vi "Write Ch 02.vi"(8 "error in":errorcluster, 10 "Producer Ch 02":T1, 11 "Chiller Cluster - 2 Channel.lvclass":refnum<class "Chiller Cluster - 2 Channel.lvclass">) -> (0 "error out":errorcluster, 3 "output cluster":refnum<class "Chiller Cluster - 2 Channel.lvclass">)   [LabVIEW 2023, in "Chiller Cluster - 2 Channel.lvclass"]
uses:
  Chiller Cluster - 2 Channel.lvclass
  Chiller Cluster - 2 Channel.lvclass/Chiller Cluster - 2 Channel.ctl
  34910d65-c21b-43eb-829c-e22e3c21e574.vi
  34910d65-c21b-43eb-829c-e22e3c21e574.vi/4bc1c15b-36ab-481f-b8dd-c64075ce723a.vi
  34910d65-c21b-43eb-829c-e22e3c21e574.vi/d83cb72b-7713-41fc-a3d1-682de79cf574.vi
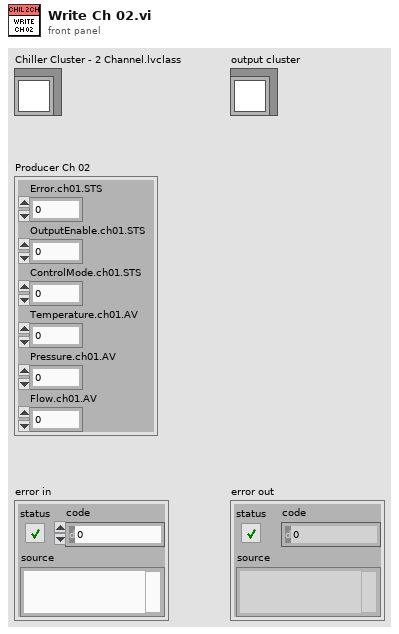
[diagram p1: front panel]
types:
  T1 = cluster{"Error.ch01.STS":i32, "OutputEnable.ch01.STS":i32, "ControlMode.ch01.STS":u16, "Temperature.ch01.AV":dbl, "Pressure.ch01.AV":dbl, "Flow.ch01.AV":dbl}
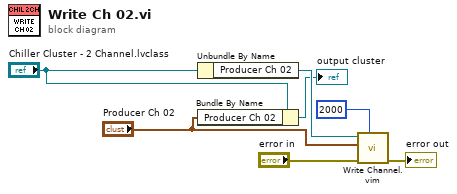
[diagram p0: block diagram]
diagram:
  n1 = Unbundle By Name("Chiller Cluster - 2 Channel.lvclass") -> ("Producer Ch 02"=w2:refnum<k21>)
  n2 = Bundle By Name(cluster="Chiller Cluster - 2 Channel.lvclass", "Producer Ch 02"="Producer Ch 02") -> (→"output cluster":refnum<class "Chiller Cluster - 2 Channel.lvclass">)
  n3 = call "Write Channel.vim"("Timeout (ms)"=2000, "error in"="error in", "Data in"="Producer Ch 02", "ADAS HIL Channel in"=w2) -> ("error out"=→"error out":errorcluster)  [unwired: 5 in, 2 out]
